vi "Acquire Data.vi"(8 "error in (no error)":errorcluster, 11 "Sensor in":refnum<class "Sensor.lvclass">) -> (0 "error out":errorcluster, 3 "Sensor out":refnum<class "Sensor.lvclass">)   [LabVIEW 2020, in "Sensor.lvclass"]
uses:
  Sensor.lvclass
  C:/Users/jharw/Documents/1 Folder to Rule them All/UMD/Inflation-Apparatus/src/Hardware/General Hardware.lvclass
  General Hardware.lvclass/General Hardware.ctl
  General Hardware.lvclass
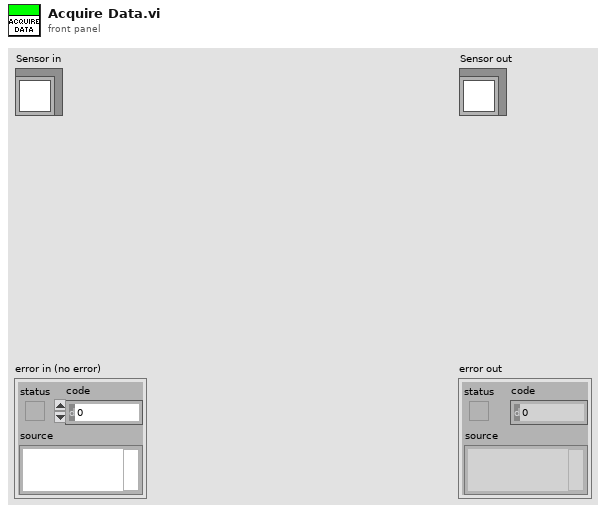
[diagram p1: front panel]
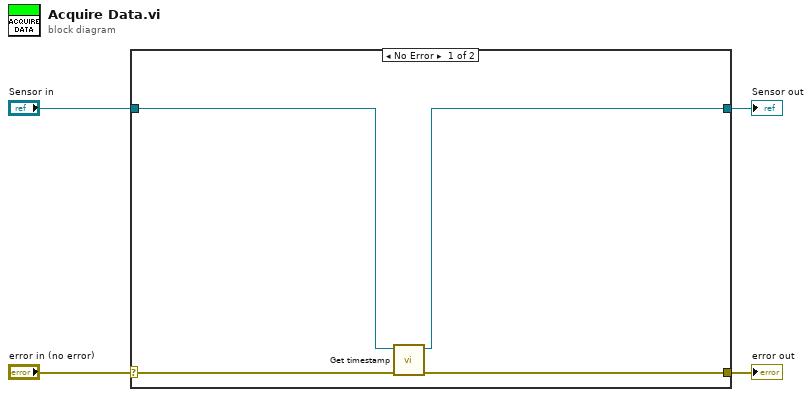
[diagram p0: block diagram]
diagram:
  n1 = case shown="No Error" "error in (no error)" {
    selector: "error in (no error)" -> [w8 w10]
    tunnel: [w7 w10] -> w3
    tunnel: [w5 w9] -> w1
    tunnel: "Sensor in" -> [w6 w9]
    frame No Error {
      n2 = call "Get timestamp.vi"("error in (no error)"=w8, "General Hardware in"=w6) -> ("error out"=w7:errorcluster, "General Hardware out"=w5:refnum<class "Sensor.lvclass">)  [unwired: 8 in]
    }
    frame Error {
    }
  }
  "error out" <- w3
  "Sensor out" <- w1
